vi "LargeScrollbar Example.vi"() -> ()   [LabVIEW 2015]
doc: "The Large Scrollbars were created initially to be used on resistive touch screen applications. Used as a QControl, events for the buttons are encapsulated and called in the Event Handler rather than being mixed with the business logic of the application.\n\nThese show an example how to create QControls with multiple controls by wrapping the controls in a cluster. Then, in the Load Reference Method change how the references are loaded and used.\n\n1. Click Run.\n2. Click Scrollbar Buttons, change the Slider or click-and-hold Scrollbar Buttons to view the different behavior.\n3. Change the maximums and try step 2 again.\n4. Click Stop to end program.\n\n<b> </b> <b> </b>\n©2016 Q Software Innovations, LLC (QSI)\nwritten by Quentin Alldredge\nproduced in LabVIEW 2015\n\nsupport@qsoftwareinnovations.com\nwww.qsoftwareinnovations.com\n\nAll rights reserved.\n\nRedistribution and use in source and binary forms, with or without modification, are permitted provided that the following conditions are met:\n\n * Redistributions of source code must retain the above copyright notice, this list of conditions and the following disclaimer.\n * Redistributions in binary form must reproduce the above copyright notice, this list of conditions and the following disclaimer in the documentation and/or other materials provided with the distribution.\n * Neither the name of Q Software Innovations, LLC. nor the names of its contributors may be used to endorse or promote products derived from this software without specific prior written permission.\n\nTHIS SOFTWARE IS PROVIDED BY THE COPYRIGHT HOLDERS AND CONTRIBUTORS \"AS IS\" AND ANY EXPRESS OR IMPLIED WARRANTIES, INCLUDING, BUT NOT LIMITED TO, THE IMPLIED WARRANTIES OF MERCHANTABILITY AND FITNESS FOR A PARTICULAR PURPOSE ARE DISCLAIMED. IN NO EVENT SHALL THE COPYRIGHT OWNER OR CONTRIBUTORS BE LIABLE FOR ANY DIRECT, INDIRECT, INCIDENTAL, SPECIAL, EXEMPLARY, OR CONSEQUENTIAL DAMAGES (INCLUDING, BUT NOT LIMITED TO, PROCUREMENT OF SUBSTITUTE GOODS OR SERVICES; LOSS OF USE, DATA, OR PROFITS; OR BUSINESS INTERRUPTION) HOWEVER CAUSED AND ON ANY THEORY OF LIABILITY, WHETHER IN CONTRACT, STRICT LIABILITY, OR TORT (INCLUDING NEGLIGENCE OR OTHERWISE) ARISING IN ANY WAY OUT OF THE USE OF THIS SOFTWARE, EVEN IF ADVISED OF THE POSSIBILITY OF SUCH DAMAGE."
uses:
  QControl Classes/LargeScrollbar/UpArrow.ctl
  QControl Classes/LargeScrollbar/DownArrow.ctl
  QControl Classes/LargeScrollbar/LeftArrow.ctl
  QControl Classes/LargeScrollbar/RightArrow.ctl
  <vilib>/Utility/miscctls.llb/LVRowAndColumnUnsignedTypeDef.ctl
  QControl Classes/LargeScrollbar/Write Max.vi
  QControl Classes/LargeScrollbar/Write Scrollbar Position.vi
  QControl Classes/LargeScrollbar/LargeScrollbar.lvclass
panel:
  in  "Stop Button":bool
  in  "Horizontal Scrollbar":T3 {"Slide" scale=0.0..4.0}
  in  "Vertical Scrollbar":T6
  in  "Data":i32(listbox)
  in  "Horizontal Scrollbar Max":u32
  in  "Vertical Scrollbar Max":u32
  out "Horizontal Scrollbar Value":u32
  out "Vertical Scrollbar Value":u32
  # "LargeScrollbars QControl Example\n\nThe Large Scrollbars were created initially to be used on resistive touch screen applications.  Used as a QControl, events for the buttons are encapsulated and called in the Event Handler rather than being mixed with the business logic of the application."
  # "These show an example how to create QControls with multiple controls by wrapping the controls in a cluster.  Then, in the Load Reference Method change how the references are loaded and used.\n\n1. Click Run.\n2. Click Scrollbar Buttons, change the Slider or click-and-hold Scrollbar Buttons to view the different behavior.\n3. Change the maximums and try step 2 again.\n4. Click Stop to end program."
  # "(Maximums are decremented by 1 to ensure last row/column remains \nvisible.  See code.)"
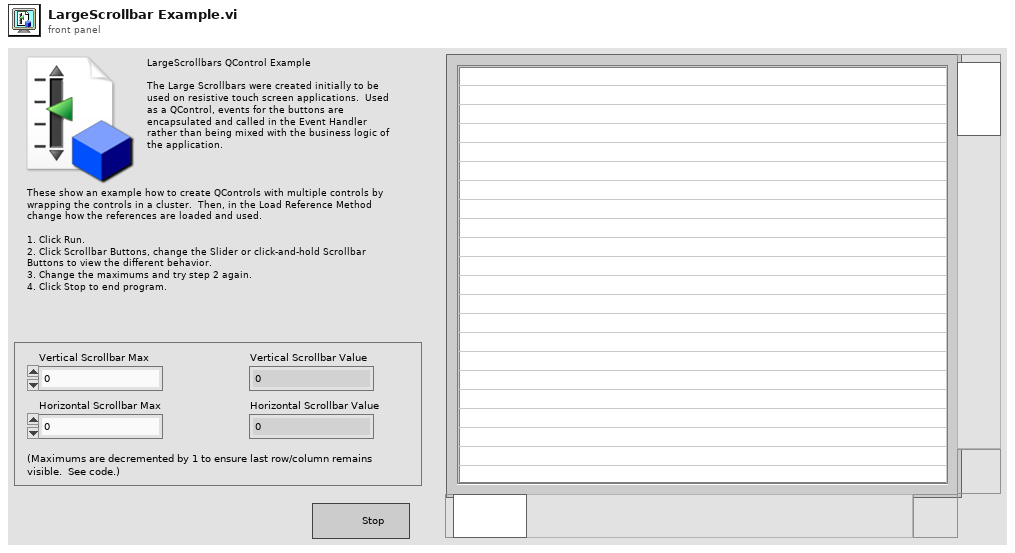
[diagram p1: front panel]
types:
  T1 = typedef "LargeScrollbar.lvclass/LeftArrow.ctl" = bool
  T2 = typedef "LargeScrollbar.lvclass/RightArrow.ctl" = bool
  T3 = cluster{"LeftButton":T1, "Slide":u32, "RightButton":T2}
  T4 = typedef "LargeScrollbar.lvclass/UpArrow.ctl" = bool
  T5 = typedef "LargeScrollbar.lvclass/DownArrow.ctl" = bool
  T6 = cluster{"UpButton":T4, "Slide":u32, "DownButton":T5}
  T7 = typedef "LVRowAndColumnUnsignedTypeDef.ctl" = cluster{"Row":u32, "Column":u32}
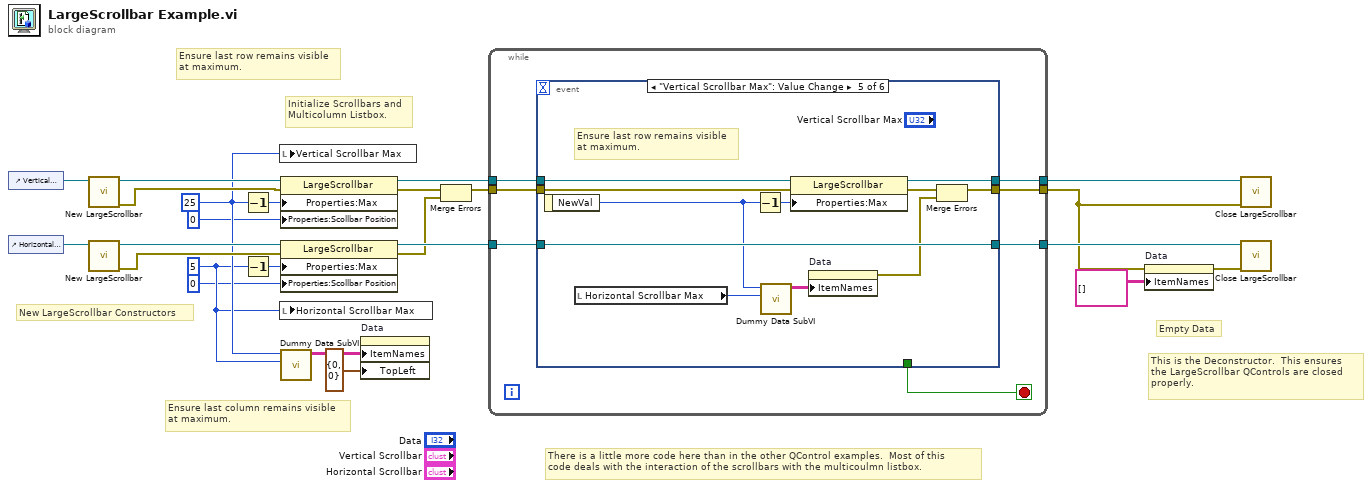
[diagram p0: block diagram]
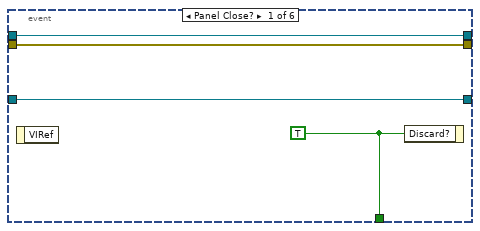
[diagram p2: hidden frame]
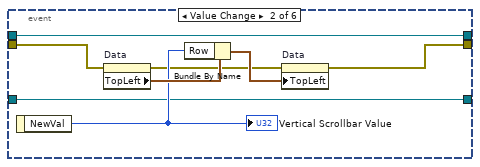
[diagram p3: hidden frame]
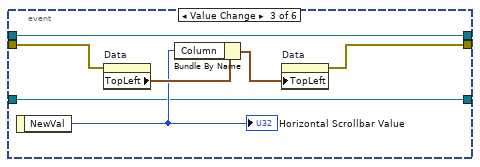
[diagram p4: hidden frame]
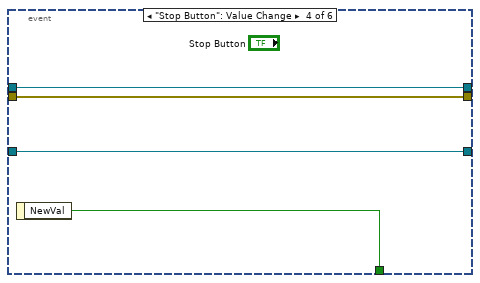
[diagram p5: hidden frame]
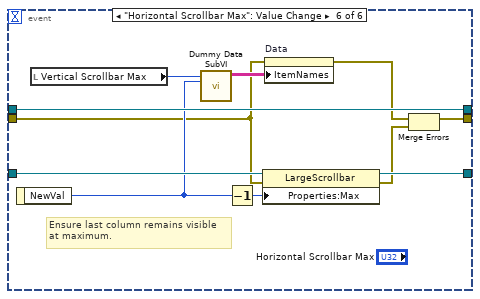
[diagram p6: hidden frame]
diagram:
  w10 = u32 5 ("Max")
  w11 = u32 25 ("Max")
  # "Empty Data"
  # "New LargeScrollbar Constructors"
  # "Ensure last column remains visible\nat maximum."
  # "Ensure last row remains visible\nat maximum."
  # "Initialize Scrollbars and \nMulticolumn Listbox."
  # "There is a little more code here than in the other QControl examples.  Most of this \ncode deals with the interaction of the scrollbars with the multicoulmn listbox."
  # "This is the Deconstructor.  This ensures \nthe LargeScrollbar QControls are closed \nproperly."
  n1 = control-ref of="Vertical Scrollbar"() -> (w24:refnum<vi>)
  n2 = control-ref of="Horizontal Scrollbar"() -> (w20:refnum<vi>)
  n3 = call "New LargeScrollbar.vi"("Reference"=w24) -> ("error out"=w16:errorcluster, "LargeScrollbar out"=w23:refnum<class "LargeScrollbar.lvclass">)  [unwired: 9 in]
  n4 = call "New LargeScrollbar.vi"("Reference"=w20) -> ("error out"=w15:errorcluster, "LargeScrollbar out"=w21:refnum<class "LargeScrollbar.lvclass">)  [unwired: 9 in]
  n5 = Decrement(x=w11) -> (x-1=w8:u32)
  n6 = Decrement(x=w10) -> (x-1=w7:u32)
  n7 = local write "Vertical Scrollbar Max"(w11) -> ()
  n8 = local write "Horizontal Scrollbar Max"(w10) -> ()
  n9 = property class="LargeScrollbar"(reference=w23, error in=w16, "Properties:Max"=w8, "Properties:Scollbar Position"=u32 0 ("Scollbar Position")) -> (reference out=w22:refnum<class "LargeScrollbar.lvclass">, error out=w14:errorcluster)
  n10 = property class="LargeScrollbar"(reference=w21, error in=w15, "Properties:Max"=w7, "Properties:Scollbar Position"=u32 0 ("Scollbar Position")) -> (reference out=w19:refnum<class "LargeScrollbar.lvclass">, error out=w13:errorcluster)
  n11 = call "Dummy Data SubVI.vi"("Number of Columns"=w10, "Number of Rows"=w11) -> ("Array"=w9:string[][])  [unwired: 9 in]
  n12 = property on="Data" class="MCListbox (strict)"("ItemNames"=w9, "TopLeft"=T7 {"Row"=0, "Column"=0} ("Top Left Visible Cell")) -> ()  [unwired: 2 in, 2 out]
  n13 = Merge Errors(w14, w13) -> (w12:errorcluster)
  n14 = while {
    tunnel: w22 -> [w31]
    tunnel: w19 -> [w29]
    tunnel: [w28] -> w18
    tunnel: [w27] -> w17
    tunnel: w12 -> [w26]
    tunnel: [w25] -> w6
    stop <- w30 stop-if-true
    n15 = event shown="[4] \"Vertical Scrollbar Max\": Value Change" {
      selector: _ -> [_ _ _ _ _ _]
      dyn-events: _ -> [_ _ _ _ _ _]
      timeout: _ -> [_ _ _ _ _ _]
      tunnel: w31 -> [w34 w40 w47 w53 w65 w75]
      tunnel: [w35 _ _ w54 _ _] -> w30
      tunnel: w29 -> [w33 w39 w46 w52 w64 w76]
      tunnel: [w34 w40 w47 w53 w63 w75] -> w28
      tunnel: [w33 w39 w46 w52 w64 w74] -> w27
      tunnel: w26 -> [w32 w38 w45 w51 w58 w69]
      tunnel: [w32 w36 w44 w51 w55 w66] -> w25
      event Panel Close? {
        w35 = TRUE ("Discard?")
        n16 = event-data() -> ()  [unwired: 1 in, 1 out]
        n17 = event-data("Discard?"=w35) -> ()  [unwired: 1 in, 1 out]
      }
      event "Vertical Scrollbar.Slide": Value Change {
        n18 = event-data() -> ("NewVal"=w42:u32)  [unwired: 1 in]
        "Vertical Scrollbar Value" <- w42
        n19 = property on="Data" class="MCListbox (strict)"(error in=w38) -> (error out=w37:errorcluster, "TopLeft"=w43:T7)  [unwired: 1 in, 1 out]
        n20 = Bundle By Name(cluster=w43, "Row"=w42) -> (w41:T7)
        n21 = property on="Data" class="MCListbox (strict)"(error in=w37, "TopLeft"=w41) -> (error out=w36:errorcluster)  [unwired: 1 in, 1 out]
      }
      event "Horizontal Scrollbar.Slide": Value Change {
        n22 = event-data() -> ("NewVal"=w48:u32)  [unwired: 1 in]
        "Horizontal Scrollbar Value" <- w48
        n23 = property on="Data" class="MCListbox (strict)"(error in=w45) -> ("TopLeft"=w50:T7)  [unwired: 1 in, 2 out]
        n24 = Bundle By Name(cluster=w50, "Column"=w48) -> (w49:T7)
        n25 = property on="Data" class="MCListbox (strict)"("TopLeft"=w49) -> (error out=w44:errorcluster)  [unwired: 2 in, 1 out]
      }
      event "Stop Button": Value Change {
        n26 = event-data() -> ("NewVal"=w54:bool)  [unwired: 1 in]
      }
      event "Vertical Scrollbar Max": Value Change {
        # "Ensure last row remains visible\nat maximum."
        n27 = event-data() -> ("NewVal"=w62:u32)  [unwired: 1 in]
        n28 = local read "Horizontal Scrollbar Max"() -> (w61:u32)
        n29 = Decrement(x=w62) -> (x-1=w59:u32)
        n30 = call "Dummy Data SubVI.vi"("Number of Columns"=w61, "Number of Rows"=w62) -> ("Array"=w60:string[][])  [unwired: 9 in]
        n31 = property class="LargeScrollbar"(reference=w65, error in=w58, "Properties:Max"=w59) -> (reference out=w63:refnum<class "LargeScrollbar.lvclass">, error out=w57:errorcluster)
        n32 = property on="Data" class="MCListbox (strict)"("ItemNames"=w60) -> (error out=w56:errorcluster)  [unwired: 2 in, 1 out]
        n33 = Merge Errors(w57, w56) -> (w55:errorcluster)
      }
      event "Horizontal Scrollbar Max": Value Change {
        # "Ensure last column remains visible\nat maximum."
        n34 = event-data() -> ("NewVal"=w72:u32)  [unwired: 1 in]
        n35 = local read "Vertical Scrollbar Max"() -> (w73:u32)
        n36 = call "Dummy Data SubVI.vi"("Number of Columns"=w72, "Number of Rows"=w73) -> ("Array"=w71:string[][])  [unwired: 9 in]
        n37 = Decrement(x=w72) -> (x-1=w70:u32)
        n38 = property class="LargeScrollbar"(reference=w76, error in=w69, "Properties:Max"=w70) -> (reference out=w74:refnum<class "LargeScrollbar.lvclass">, error out=w68:errorcluster)
        n39 = property on="Data" class="MCListbox (strict)"(error in=w69, "ItemNames"=w71) -> (error out=w67:errorcluster)  [unwired: 1 in, 1 out]
        n40 = Merge Errors(w67, w68) -> (w66:errorcluster)
      }
    }
  }
  n41 = property on="Data" class="MCListbox (strict)"(error in=w6, "ItemNames"=string[][] [] ("Item Names")) -> (error out=w5:errorcluster)  [unwired: 1 in, 1 out]
  n42 = call "Close LargeScrollbar.vi"("error in (no error)"=w6, "LargeScrollbar in"=w18) -> ()  [unwired: 8 in, 2 out]
  n43 = call "Close LargeScrollbar.vi"("error in (no error)"=w5, "LargeScrollbar in"=w17) -> ()  [unwired: 8 in, 2 out]
